vi "send email.vi"(7 "Body text":string, 8 "error in (no error)":errorcluster, 9 "Email settings":T1, 10 "Jpeg":path, 11 "Data":path) -> (0 "error out":errorcluster)   [LabVIEW 2014]
uses:
  <vilib>/smtpClient/Set Message Text.vi
  <vilib>/smtpClient/LabVIEWSMTPClient.lvlib
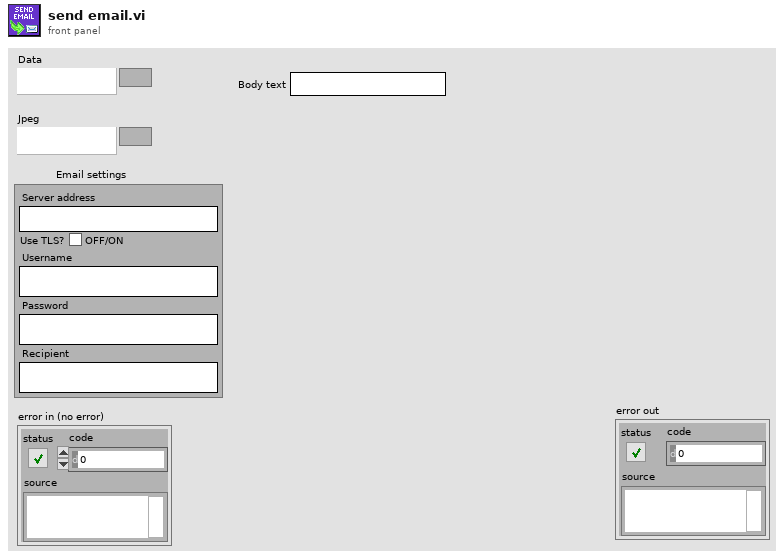
[diagram p1: front panel]
types:
  T1 = cluster{"Server address":string, "Use TLS?":bool, "Username":string, "Password":string, "Recipient":string}
  T2 = typedef "LabVIEWSMTPClient.lvlib/SmtpClientHandle.ctl" = refnum<k1>
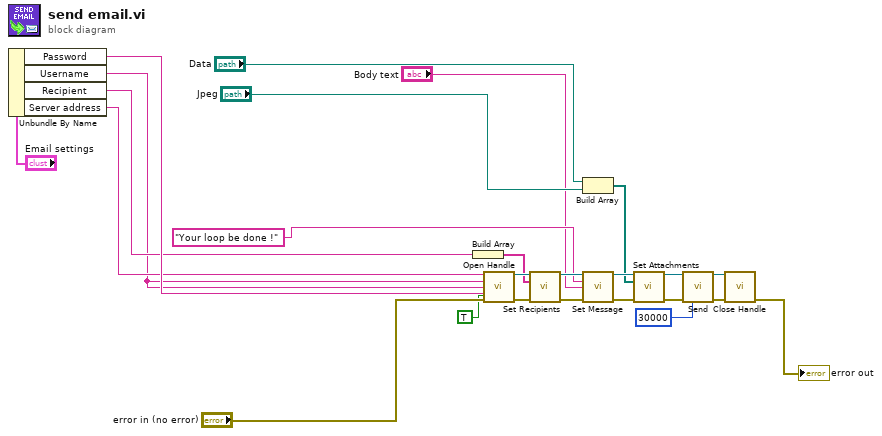
[diagram p0: block diagram]
diagram:
  n1 = Unbundle By Name("Email settings") -> ("Password"=w5:string, "Username"=w2:string, "Recipient"=w3:string, "Server address"=w4:string)
  n2 = Build Array(w3) -> (w6:string[])
  n3 = call <vilib>:"Open Handle.vi"("server address"=w4, "from"=w2, "username"=w2, "password"=w5, "error in (no error)"="error in (no error)", "use TLS (false)"=TRUE) -> ("handle out"=w23:T2, "error out"=w22:errorcluster)  [unwired: 8 in]
  n4 = call <vilib>:"Set Recipients.vi"("handle in"=w23, "to"=w6, "error in (no error)"=w22) -> ("handle out"=w21:T2, "error out"=w20:errorcluster)  [unwired: 11 in]
  n5 = Build Array("Data", "Jpeg") -> (w11:path[])
  n6 = call-poly <vilib>:"Set Message.vi"("handle in"=w21, "subject"="Your loop be done !", "plain text message"="Body text", "error in (no error)"=w20) -> ("handle out"=w16:T2, "error out"=w14:errorcluster)  [unwired: 10 in]
  n7 = call <vilib>:"Set Attachments.vi"("handle in"=w16, "attachments"=w11, "error in (no error)"=w14) -> ("handle out"=w15:T2, "error out"=w13:errorcluster)  [unwired: 11 in]
  n8 = call <vilib>:"Send.vi"("handle in"=w15, "error in (no error)"=w13, "timeout in ms (10000)"=30000) -> ("handle out"=w19:T2, "error out"=w18:errorcluster)  [unwired: 10 in, 1 out]
  n9 = call <vilib>:"Close Handle.vi"("handle in"=w19, "error in (no error)"=w18) -> ("error out"=→"error out":errorcluster)  [unwired: 12 in, 1 out]
